vi "Dodanie wskazanego punktu z listy współrzędnych do mapy.vi"(6 "Właściwości punktów z listy":T1, 8 "Lista współrzędnych":string[][](array[string]), 9 "Nr punktu":i16, 10 "Długość piksela w metrach":dbl, 11 "Mapa terenu":picture) -> (3 "Mapa z wprowadzonym punktem":picture)   [LabVIEW 2015, in "Biblioteka moduł map v3.lvlib" / "Obsługa grafiki mapy.lvlib"]
uses:
  Pomocnicze/Pomocnicze.lvlib
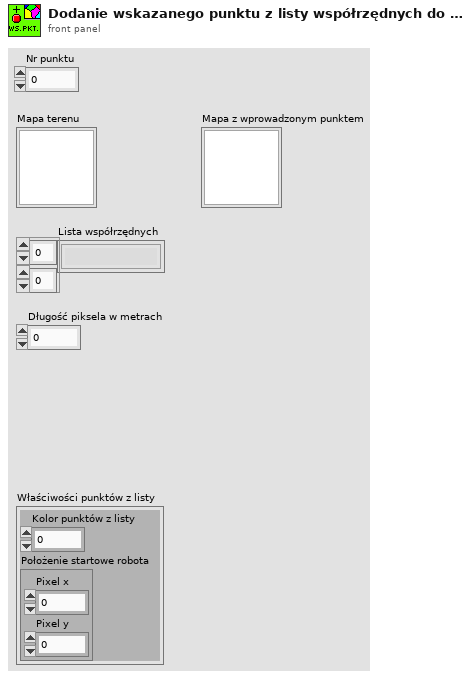
[diagram p1: front panel]
types:
  T1 = cluster{"Kolor punktów z listy":u32, "Położenie startowe robota":cluster{"Pixel x":i16, "Pixel y":i16}}
  T2 = cluster{"Położenie":cluster{"Pixel x":i16, "Pixel y":i16}, "Kolor punktu":u32, "Rozmiar punktu":u32, "Nazwa punktu":string}
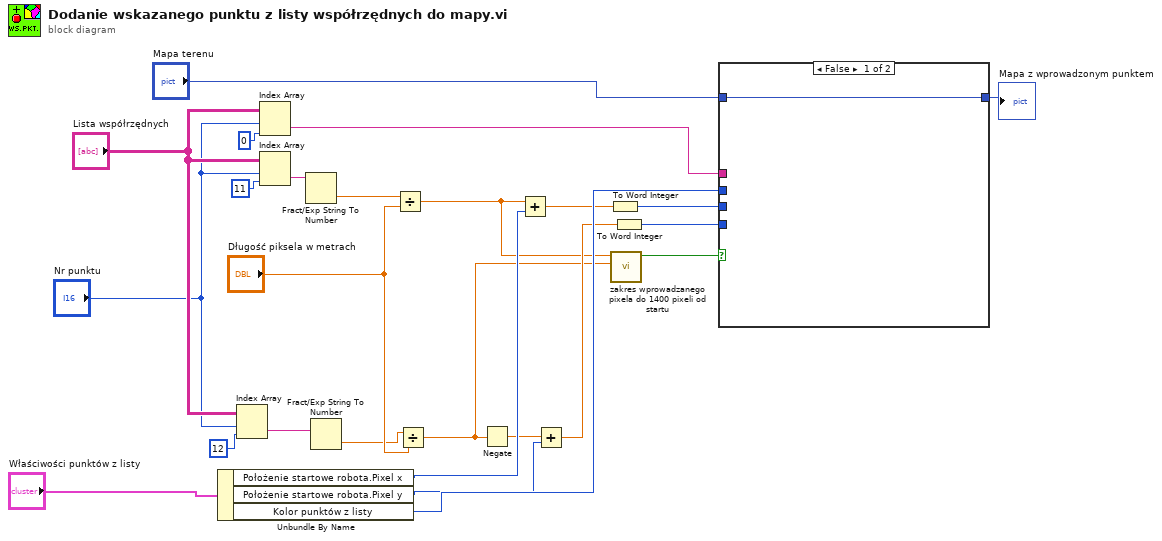
[diagram p0: block diagram]
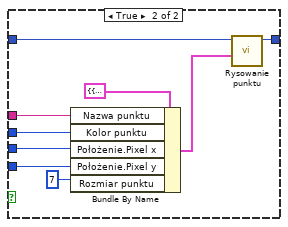
[diagram p2: hidden frame]
diagram:
  n1 = Unbundle By Name("Właściwości punktów z listy") -> ("Położenie startowe robota.Pixel x"=w22:i16, "Położenie startowe robota.Pixel y"=w23:i16, "Kolor punktów z listy"=w24:u32)
  n2 = Index Array(array="Lista współrzędnych", index (row)="Nr punktu", index (col)=12 ("disabled index (col)")) -> (element=w16:string)
  n3 = Index Array(array="Lista współrzędnych", index (row)="Nr punktu", index (col)=0 ("disabled index (col)")) -> (element=w17:string)
  n4 = Index Array(array="Lista współrzędnych", index (row)="Nr punktu", index (col)=11 ("disabled index (col)")) -> (element=w11:string)
  n5 = Fract/Exp String To Number(string=w11) -> (number=w18:dbl)  [unwired: 3 in, 1 out]
  n6 = Fract/Exp String To Number(string=w16) -> (number=w20:dbl)  [unwired: 3 in, 1 out]
  n7 = Divide(x=w18, y="Długość piksela w metrach") -> (x/y=w3:dbl)
  n8 = Divide(x=w20, y="Długość piksela w metrach") -> (x/y=w2:dbl)
  n9 = Negate(x=w2) -> (-x=w19:dbl)
  n10 = Add(x=w3, y=w22) -> (x+y=w6:dbl)
  n11 = Add(x=w19, y=w23) -> (x+y=w5:dbl)
  n12 = To Word Integer(number=w6) -> (16bit integer=w4:i16)
  n13 = call "zakres wprowadzanego pixela do 1400 pixeli od startu.vi"("Numeric 2"=w2, "Numeric"=w3) -> ("Boolean"=w1:bool)  [unwired: 9 in]
  n14 = To Word Integer(number=w5) -> (16bit integer=w7:i16)
  n15 = case shown="False" w1 {
    tunnel: w24 -> [_ w35]
    tunnel: w17 -> [_ w33]
    tunnel: [w26 w30] -> w13
    tunnel: "Mapa terenu" -> [w26 w29]
    tunnel: w7 -> [_ w28]
    tunnel: w4 -> [_ w27]
    frame False {
    }
    frame True {
      n16 = Bundle By Name(cluster=T2 {"Położenie"={"Pixel x"=0, "Pixel y"=0}, "Kolor punktu"=0, "Rozmiar punktu"=2, "Nazwa punktu"=""} ("Punkt na mapie"), "Nazwa punktu"=w33, "Kolor punktu"=w35, "Położenie.Pixel x"=w27, "Położenie.Pixel y"=w28, "Rozmiar punktu"=u32 7) -> (w32:T2)
      n17 = call "Rysowanie punktu.vi"("Punkt na mapie"=w32, "Mapa terenu"=w29) -> ("Mapa z wprowadzonym punktem"=w30:picture)  [unwired: 9 in]
    }
  }
  "Mapa z wprowadzonym punktem" <- w13
